vi "GOH.vi"(0 "System no.":i32=1 min=1 max=4 step=1, 2 "GOH axes":string[](array[string]), 3 "All axes?":bool, 4 "Axis identifier?":bool=TRUE, 5 "error in":errorcluster) -> (19 "error out":errorcluster)   [LabVIEW 2020]
doc: "Moves specified axes to their home positions.\n\nC-702, C-843, C-843.PM, C-844, C-848, C-865, C-866, C-867,C-877,C-880, E-710, E-861, E-871, E-873, E-874, Mercury_GCS: If All axes? = TRUE, then Axis identifier? must be TRUE\n\nC-880K005: VI only supported when called through PI_Multix.vi\n\nE-755: If All axes? = TRUE, then Axis identifier? can be FALSE. Command not available for E-755.101.\n\nE-517, E-518, E-761, Mercury: If All axes? = TRUE, then Axis identifier? can be FALSE"
panel:
  # "Moves specified axes to their home positions."
  # "If all axes: use"
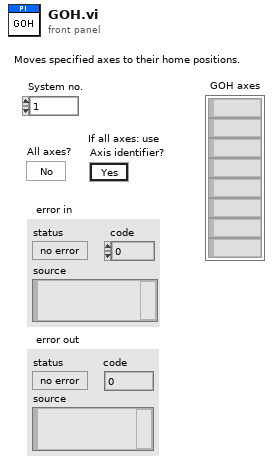
[diagram p1: front panel]
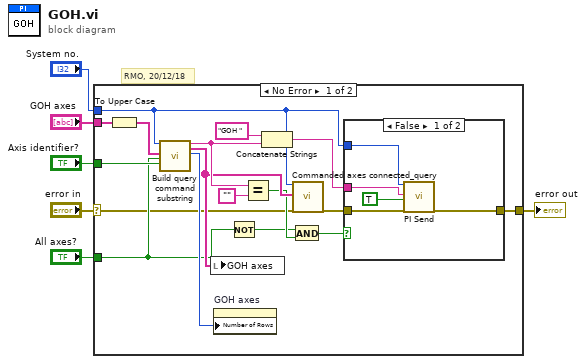
[diagram p0: block diagram]
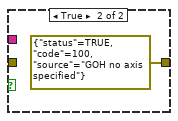
[diagram p2: hidden frame]
diagram:
  # "RMO, 20/12/18"
  n1 = case shown="No Error" "error in" {
    selector: "error in" -> [w7 w30]
    tunnel: "GOH axes" -> [w22 _]
    tunnel: "Axis identifier?" -> [w19 _]
    tunnel: "System no." -> [w8 _]
    tunnel: "All axes?" -> [w14 _]
    tunnel: [w11 w30] -> w2
    frame No Error {
      n2 = To Upper Case(1:w22) -> (0:w20:string[])
      n3 = call "Build query command substring.vi"("System no."=w8, "Axes to query in"=w20, "Query\nAll axes?"=w14, "For all axes: use\nAxis identifier?"=w19) -> ("Command substring"=w18:string, "Axes to query out"=w17:string[], "Number of rows"=w16:u32)  [unwired: 2 in, 11 out]
      n4 = local write "GOH axes"(w17) -> ()
      n5 = property on="GOH axes" class="Arr (strict)"("Number of Rows"=w16) -> ()  [unwired: 2 in, 2 out]
      n6 = Not(x=w14) -> (.not. x?=w13:bool)
      n7 = Equal?(x=w18, y="" ("x")) -> (x = y?=w15:bool)
      n8 = Concatenate Strings("GOH ", w18) -> (w9:string)
      n9 = And(x=w13, y=w15) -> (x .and. y?=w12:bool)
      n10 = call "Commanded axes connected_query.vi"("System no."=w8, "Commanded axes"=w17, "error in"=w7) -> ("error out"=w10:errorcluster)  [unwired: 1 in, 15 out]
      n11 = case shown="False" w12 {
        tunnel: [w24 errorcluster {"status"=TRUE, "code"=100, "source"="GOH no axis specified"} ("error out")] -> w11
        tunnel: w10 -> [w28 _]
        tunnel: w9 -> [w26 _]
        tunnel: w8 -> [w25 _]
        frame False {
          n12 = call "PI Send.vi"("System no."=w25, "String to send"=w26, "Attach termination char.?"=TRUE ("Attach Linefeed?"), "error in"=w28) -> ("error out"=w24:errorcluster)  [unwired: 2 in, 13 out]
        }
        frame True {
        }
      }
    }
    frame Error {
    }
  }
  "error out" <- w2
